vi "LDA_IP_An_mx.vi"(0 "Board type":T1=enum."NI-DAQmx", 1 "interval scanning":bool, 7 "Trigger mode":T2, 9 "output polarity":u16(ring)=1 items=["do not change", "positive", "negative"], 13 "Local Client?":bool=TRUE) -> (3 "LDA Binary output":u16[][](array[numeric]), 6 "I16 TOF block (mu.s)":i16[](array[numeric])=[-338, -324, -346, -351, -326, -357, -344, -311, -375, -296], 15 "error out":errorcluster)   [LabVIEW 2011]
uses:
  Controls/Trigger_Mode.ctl
  Controls/Board_Types.ctl
  Controls/Block_start_and_end.ctl
  <vilib>/DAQmx/read.llb/DAQmx Read (Analog 2D DBL NChan NSamp).vi
  Globals/Meas_global.vi
  Globals/LDA_meas_global_1.vi
  PWA/PWAtasksGLOBAL.vi
  <vilib>/DAQmx/configure/timing.llb/DAQmx Timing (Sample Clock).vi
  <vilib>/DAQmx/create/channels.llb/DAQmx Create Channel (AI-Voltage-Basic).vi
  Globals/LDA_meas_global_2.vi
  <vilib>/DAQmx/miscellaneous.llb/DAQmx Fill In Error Info.vi
  Program Files/National Instruments/LabVIEW 2011/resource/objmgr/daqmx.rc
panel:
  out "AI.Voltage.Rngs":dbl[](array[numeric])=[-10.0, 10.0]
  out "TotalSampPerChanAcquired":dbl=1024.0
  out "AvailSampPerChan":u32
  out "CurrReadPos":dbl=1024.0
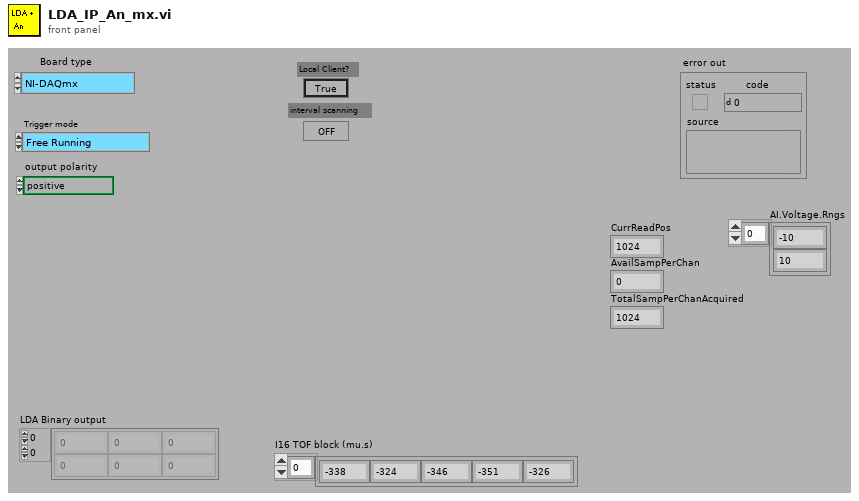
[diagram p1: front panel]
types:
  T1 = typedef "Board_Types.ctl" = enum16{"Simulate", "Local ADAM", "Server ADAM", "NI-DAQmx", "NI-DAQmxBase", "ADC488", "DT LV-link"}
  T2 = typedef "Trigger_Mode.ctl" = enum16{"Free Running", "Start on Trigger", "Trigger Every Block", "Trigger Every Sample"}
  T3 = typedef "Ch_and_Spans.ctl" = cluster{"high limit (10V)":sgl, "low limit (-10V)":sgl, "Ch No":i16, "Var name":string, "Use Latest Calib":bool}
  T4 = typedef "Block_start_and_end.ctl" = cluster{"Started":dbl, "Ended":dbl, "Analogue Frequency Hz":dbl}
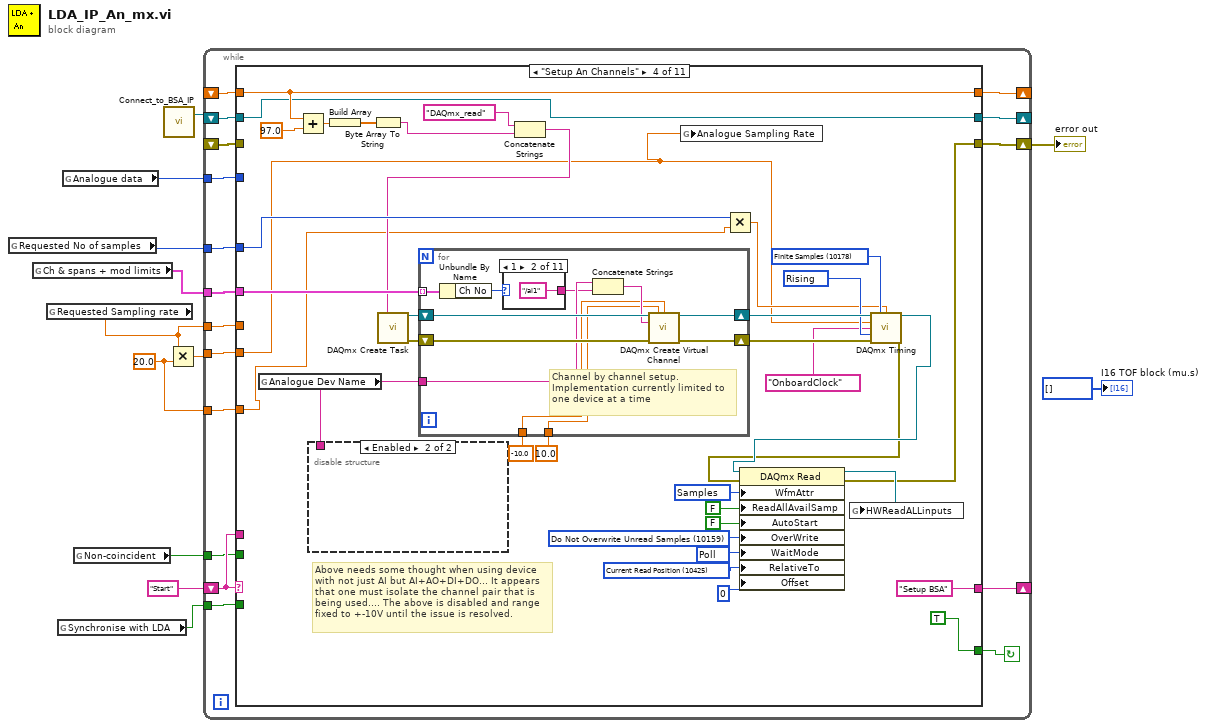
[diagram p0: block diagram]
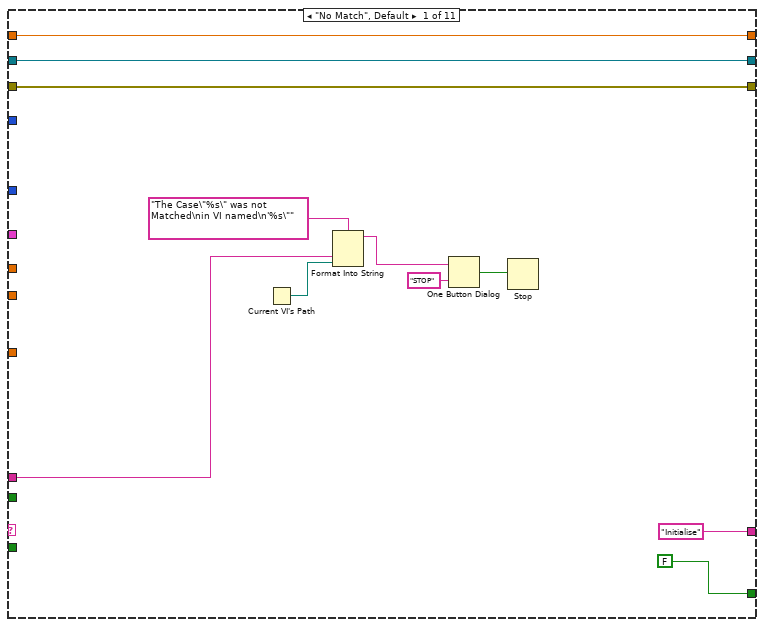
[diagram p2: hidden frame]
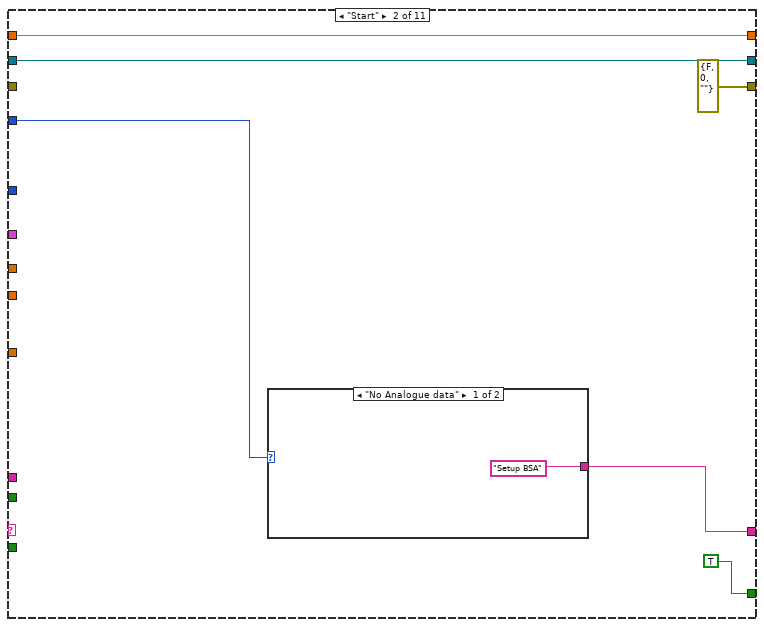
[diagram p3: hidden frame]
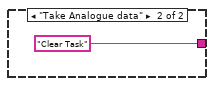
[diagram p4: hidden frame]
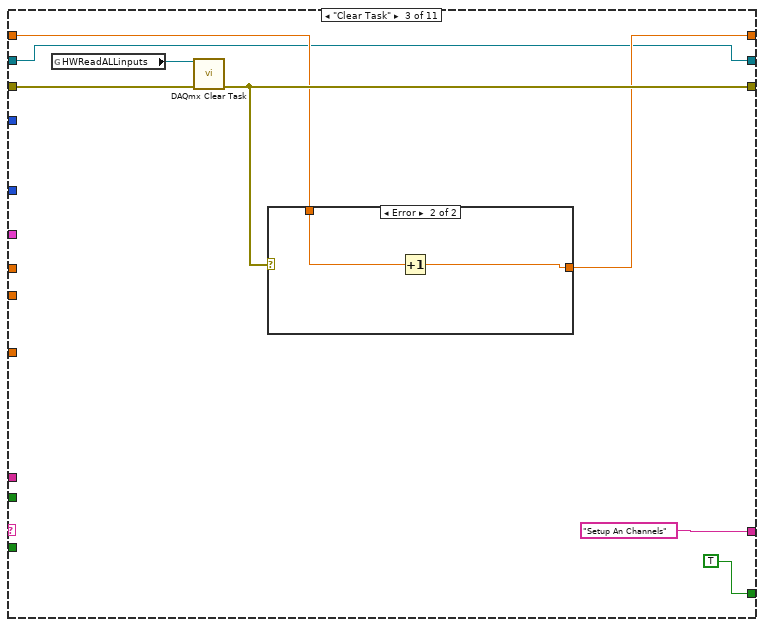
[diagram p5: hidden frame]
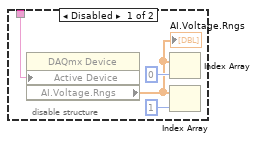
[diagram p7: hidden frame]
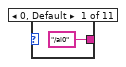
[diagram p8: hidden frame]
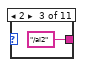
[diagram p9: hidden frame]
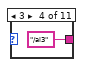
[diagram p10: hidden frame]
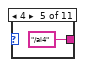
[diagram p11: hidden frame]
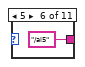
[diagram p12: hidden frame]
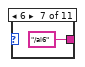
[diagram p13: hidden frame]
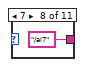
[diagram p14: hidden frame]
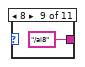
[diagram p15: hidden frame]
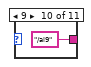
[diagram p16: hidden frame]
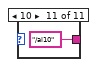
[diagram p17: hidden frame]
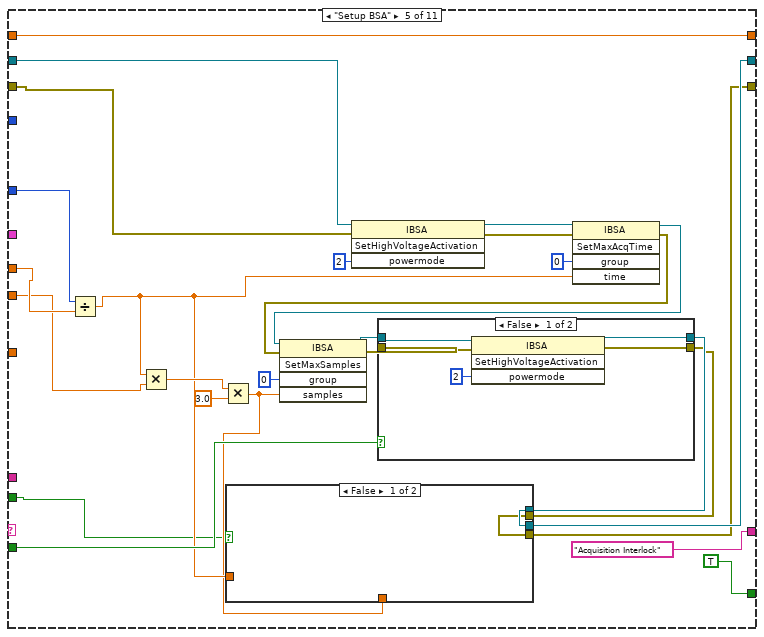
[diagram p18: hidden frame]
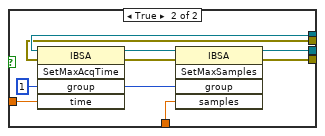
[diagram p19: hidden frame]
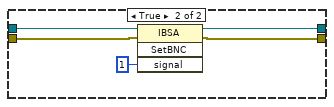
[diagram p20: hidden frame]
diagram:
  w8 = 20.0 ("y")
  n1 = global read "Meas_global.vi" "Requested No of samples"() -> (w1:i32)
  n2 = global read "Meas_global.vi" "Ch & spans + mod limits"() -> (w3:T3[])
  n3 = global read "Meas_global.vi" "Requested Sampling rate"() -> (w2:dbl)
  n4 = global read "Meas_global.vi" "Synchronise with LDA"() -> (w5:bool)
  n5 = global read "Meas_global.vi" "Analogue data"() -> (w6:enum16{"No Analogue data", "Take Analogue data"})
  n6 = global read "LDA_meas_global_1.vi" "Non-coincident"() -> (w4:bool)
  n7 = call "Connect_to_BSA_IP.vi"() -> ("BSA"=w7:refnum<k7>)  [unwired: 3 out]
  n8 = Multiply(x=w2, y=w8) -> (x*y=w9:dbl)
  n9 = while {
    shift-left: "Start" -> [w27]
    shift-right: [w28] -> _
    shift-right: [w22] -> w11
    shift-left: _ -> [w26]
    tunnel: w9 -> [w25]
    tunnel: w1 -> [w24]
    tunnel: w3 -> [w23]
    shift-right: [w21] -> _
    shift-left: _ -> [w20]
    tunnel: w2 -> [w19]
    tunnel: w8 -> [w18]
    shift-right: [w16] -> _
    shift-left: w7 -> [w17]
    tunnel: w6 -> [w15]
    tunnel: w5 -> [w14]
    tunnel: w4 -> [w13]
    stop <- w29 continue-if-true
    n10 = case shown="\"Setup An Channels\"" w27 {
      tunnel: [FALSE TRUE TRUE TRUE TRUE TRUE TRUE w220 w297 FALSE FALSE] -> w29
      tunnel: ["Initialise" w44 "Setup An Channels" "Setup BSA" "Acquisition Interlock" "Start Task" w177 w241 w300 "End" "End" ("f")] -> w28
      tunnel: w27 -> [w35 _ _ _ _ _ _ _ _ _ _]
      tunnel: [w32 errorcluster {"status"=FALSE, "code"=0, "source"=""} ("error out") w52 w61 w125 w173 w191 w218 w266 w316 w325] -> w22
      tunnel: w26 -> [w32 _ w53 _ w135 w173 w179 w219 w264 w322 w325]
      tunnel: w25 -> [_ _ _ w60 w136 _ w187 _ _ _ _]
      tunnel: w24 -> [_ _ _ w87 w138 _ w189 _ _ w307 _]
      tunnel: w23 -> [_ _ _ w90 _ _ _ _ _ _ _]
      tunnel: [w31 w42 w51 w75 w134 w171 w192 w240 w299 w311 w324] -> w21
      tunnel: w20 -> [w31 w42 w50 w75 w134 w171 w192 w240 w299 w311 w324]
      tunnel: w19 -> [_ _ _ _ w137 _ w188 _ _ _ _]
      tunnel: w18 -> [_ _ _ w74 _ _ _ _ _ w310 _]
      tunnel: w17 -> [w30 w46 w49 w73 w139 w170 w185 w226 w265 w308 w323]
      tunnel: [w30 w46 w49 w73 w127 w170 w184 w214 w263 w308 w323] -> w16
      tunnel: w15 -> [_ w45 _ _ _ _ w178 w221 w298 _ _]
      tunnel: w14 -> [_ _ _ _ w129 _ _ _ _ _ _]
      tunnel: w13 -> [_ _ _ _ w122 _ w176 _ _ _ _]
      frame "No Match", Default {
        n11 = Current VI's Path() -> (path=w34:path)
        n12 = Format Into String(format string="The Case\"%s\" was not Matched\nin VI named\n'%s\"" ("Format String"), w35, w34) -> (resulting string=w38:string)  [unwired: 2 in, 1 out]
        n13 = One Button Dialog(message=w38, button name ("OK")="STOP") -> (true=w36:bool)
        n14 = Stop(stop? (T)=w36) -> ()
      }
      frame "Start" {
        n15 = case shown="\"No Analogue data\"" w45 {
          tunnel: ["Setup BSA" "Clear Task"] -> w44
          frame "No Analogue data" {
          }
          frame "Take Analogue data" {
          }
        }
      }
      frame "Clear Task" {
        n16 = global read "PWAtasksGLOBAL.vi" "HWReadALLinputs"() -> (w54:refnum<k21>)
        n17 = call <vilib>:"DAQmx Clear Task.vi"("task in"=w54, "error in"=w53) -> ("error out"=w52:errorcluster)  [unwired: 13 out]
        n18 = case shown="Error" w52 {
          tunnel: [w57 w58] -> w51
          tunnel: w50 -> [w57 w59]
          frame No Error {
          }
          frame Error {
            n19 = Increment(x=w59) -> (x+1=w58:dbl)
          }
        }
      }
      frame "Setup An Channels" {
        w66 = 10425 items=["First Sample"=10424, "Current Read Position"=10425, "Reference Trigger"=10426, "First Pretrigger Sample"=10427, "Most Recent Sample"=10428] ("RelativeTo")
        w67 = 12524 items=["Wait For Interrupt"=12523, "Poll"=12524, "Yield"=12525, "Sleep"=12547] ("WaitMode")
        w68 = 10159 items=["Overwrite Unread Samples"=10252, "Do Not Overwrite Unread Samples"=10159] ("OverWrite")
        w70 = 10287 items=["Samples"=10287, "Samples and Timing"=10140, "Samples, Timing, and Attributes"=10141] ("WfmAttr")
        w89 = 10280 items=["Rising"=10280, "Falling"=10171] ("active edge")
        w93 = 10178 items=["Finite Samples"=10178, "Continuous Samples"=10123, "Hardware Timed Single Point"=12522] ("sample mode")
        # "Above needs some thought when using device with not just AI but AI+AO+DI+DO... It appears that one must isolate the channel pair that is being used.... The above is disabled and range fixed to +-10V until the issue is resolved."
        n20 = global read "PWAtasksGLOBAL.vi" "Analogue Dev Name"() -> (w82:string)
        n21 = Add(x=w75, y=97.0) -> (x+y=w80:dbl)
        n22 = disable-structure shown="Enabled" {
          disable-tunnel: w82 -> [w96 _]
          frame Disabled {
            n23 = property class="DAQmx Device"("Active Device"=w96) -> ("AI.Voltage.Rngs"=w97:dbl[])  [unwired: 2 in, 2 out]
            "AI.Voltage.Rngs" <- w97
            n24 = Index Array(array=w97, index=0) -> ()  [unwired: 1 out]
            n25 = Index Array(array=w97, index=1) -> ()  [unwired: 1 out]
          }
          frame Enabled {
          }
        }
        n26 = Build Array(w80) -> (w79:dbl[])
        n27 = Byte Array To String(unsigned byte array=w79) -> (string=w77:string)
        n28 = Concatenate Strings("DAQmx_read" ("new task name"), w77) -> (w76:string)
        n29 = call <vilib>:"DAQmx Create Task.vi"("new task name"=w76) -> ("task out"=w91:refnum<k21>, "error out"=w94:errorcluster)  [unwired: 4 in, 9 out]
        n30 = for {
          tunnel: w90 -> [w110] mode=indexing
          shift-right: [w108] -> w92
          shift-left: w91 -> [w109]
          shift-right: [w106] -> w95
          shift-left: w94 -> [w107]
          tunnel: w82 -> [w104]
          tunnel: -10.0 -> [w101]
          tunnel: 10.0 -> [w100]
          # "Channel by channel setup. Implementation currently limited to one device at a time"
          n31 = Unbundle By Name(w110) -> ("Ch No"=w105:i16)
          n32 = case shown="1" w105 {
            tunnel: ["/ai0" ("string") "/ai1" ("string") "/ai2" ("string") "/ai3" ("string") "/ai4" ("string") "/ai5" ("string") "/ai6" ("string") "/ai7" ("string") "/ai8" ("string") "/ai9" ("string") "/ai10" ("string")] -> w103
            frame 0, Default {
            }
            frame 1 {
            }
            frame 2 {
            }
            frame 3 {
            }
            frame 4 {
            }
            frame 5 {
            }
            frame 6 {
            }
            frame 7 {
            }
            frame 8 {
            }
            frame 9 {
            }
            frame 10 {
            }
          }
          n33 = Concatenate Strings(w104, w103) -> (w102:string)
          n34 = call-poly <vilib>:"DAQmx Create Virtual Channel.vi"("task in"=w109, "maximum value"=w100, "minimum value"=w101, "physical channels"=w102, "error in"=w107) -> ("task out"=w108:refnum<k21>, "error out"=w106:errorcluster)  [unwired: 4 in, 5 out]
        }
        n35 = global write "Meas_global.vi" "Analogue Sampling Rate"(w60) -> ()
        n36 = Multiply(x=w87, y=w74) -> (x*y=w86:dbl)
        n37 = call-poly <vilib>:"DAQmx Timing.vi"("task/channels in"=w92, "sample mode"=w93, "samples per channel"=w86, "rate"=w60, "source"=tag "OnboardClock", "active edge"=w89, "error in"=w95) -> ("task out"=w64:refnum<k21>, "error out"=w62:errorcluster)  [unwired: 7 out]
        n38 = property class="DAQmx Read"(reference=w64, error in=w62, "WfmAttr"=w70, "ReadAllAvailSamp"=FALSE, "AutoStart"=FALSE, "OverWrite"=w68, "WaitMode"=w67, "RelativeTo"=w66, "Offset"=0) -> (reference out=w63:refnum<k21>, error out=w61:errorcluster)
        n39 = global write "PWAtasksGLOBAL.vi" "HWReadALLinputs"(w63) -> ()
      }
      frame "Setup BSA" {
        n40 = Divide(x=w138, y=w137) -> (x/y=w124:dbl)
        n41 = Multiply(x=w124, y=w136) -> (x*y=w140:dbl)
        n42 = Multiply(x=w140, y=3.0) -> (x*y=w123:dbl)
        n43 = invoke class="IBSA" method="SetHighVoltageActivation"(reference=w139, error in=w135, "powermode"=2) -> (reference out=w146:refnum<k7>, error out=w148:errorcluster)  [unwired: 1 in, 2 out]
        n44 = invoke class="IBSA" method="SetMaxAcqTime"(reference=w146, error in=w148, "group"=0, "time"=w124) -> (reference out=w147:refnum<k7>, error out=w145:errorcluster)  [unwired: 1 in, 3 out]
        n45 = invoke class="IBSA" method="SetMaxSamples"(reference=w147, error in=w145, "group"=0, "samples"=w123) -> (reference out=w131:refnum<k7>, error out=w130:errorcluster)  [unwired: 1 in, 3 out]
        n46 = case shown="False" w129 {
          tunnel: w131 -> [w163 w168]
          tunnel: w130 -> [w162 w167]
          tunnel: [w161 w166] -> w128
          tunnel: [w160 w165] -> w126
          frame False {
            n47 = invoke class="IBSA" method="SetHighVoltageActivation"(reference=w163, error in=w162, "powermode"=2) -> (reference out=w161:refnum<k7>, error out=w160:errorcluster)  [unwired: 1 in, 2 out]
          }
          frame True {
            n48 = invoke class="IBSA" method="SetBNC"(reference=w168, error in=w167, "signal"=1) -> (reference out=w166:refnum<k7>, error out=w165:errorcluster)  [unwired: 1 in, 2 out]
          }
        }
        n49 = case shown="False" w122 {
          tunnel: w128 -> [w150 w157]
          tunnel: [w150 w155] -> w127
          tunnel: w126 -> [w149 w154]
          tunnel: [w149 w153] -> w125
          tunnel: w124 -> [_ w152]
          tunnel: w123 -> [_ w151]
          frame False {
          }
          frame True {
            w158 = 1 ("group")
            n50 = invoke class="IBSA" method="SetMaxAcqTime"(reference=w157, error in=w154, "group"=w158, "time"=w152) -> (reference out=w156:refnum<k7>, error out=w159:errorcluster)  [unwired: 1 in, 3 out]
            n51 = invoke class="IBSA" method="SetMaxSamples"(reference=w156, error in=w159, "group"=w158, "samples"=w151) -> (reference out=w155:refnum<k7>, error out=w153:errorcluster)  [unwired: 1 in, 3 out]
          }
        }
      }
      frame "Acquisition Interlock" {
        n52 = call "Acquisition_Interlock.vi"("Local Control"="Local Client?") -> ()
      }
      frame "Start Task" {
        n53 = Divide(x=w189, y=w188) -> (x/y=w186:dbl)
        n54 = global read "PWAtasksGLOBAL.vi" "HWReadALLinputs"() -> (w180:refnum<k21>)
        n55 = Multiply(x=w186, y=w187) -> (x*y=w183:dbl)
        n56 = Multiply(x=w183, y=3.0) -> (x*y=w182:dbl)
        n57 = case shown="\"Take Analogue data\"" w178 {
          tunnel: w179 -> [w199 w206]
          tunnel: [w198 w204] -> w191
          tunnel: w180 -> [w200 w208]
          tunnel: [w200 w207] -> w190
          tunnel: w186 -> [_ _]
          tunnel: w182 -> [_ _]
          tunnel: w185 -> [w196 w205]
          tunnel: [w197 w203] -> w184
          frame "No Analogue data" {
            n58 = invoke class="IBSA" method="StartAcq"(reference=w196, error in=w199, "waitAcqDone"=1) -> (reference out=w197:refnum<k7>, error out=w198:errorcluster)  [unwired: 1 in, 2 out]
          }
          frame "Take Analogue data" {
            n59 = stacked-sequence {
              tunnel: w208 -> [_ w211]
              tunnel: [_ w210] -> w207
              frame #0 {
                n60 = Wait (ms)(milliseconds to wait=u32 600) -> ()  [unwired: 1 out]
              }
              frame #1 {
                n61 = call <vilib>:"DAQmx Start Task.vi"("task/channels in"=w211) -> ("task out"=w210:refnum<k21>)  [unwired: 1 in, 13 out]
              }
            }
            n62 = invoke class="IBSA" method="StartAcq"(reference=w205, error in=w206, "waitAcqDone"=1) -> (reference out=w203:refnum<k7>, error out=w204:errorcluster)  [unwired: 1 in, 2 out]
          }
        }
        n63 = case shown="True" w176 {
          tunnel: ["Get LDA Data" "Get LDA data Non-coincident"] -> w177
          frame False {
          }
          frame True {
          }
        }
        n64 = global write "PWAtasksGLOBAL.vi" "HWReadALLinputs"(w190) -> ()
      }
      frame "Get LDA Data" {
        w234 = dbl[] []  # Array Constant
        w222 = 0 ("group")
        n65 = invoke class="IBSA" method="ReadArrivalTimeData"(reference=w226, error in=w219, "group"=w222) -> (reference out=w239:refnum<k7>, error out=w238:errorcluster, "ReadArrivalTimeData"=w233:variant)  [unwired: 1 in, 1 out]
        n66 = global read "Meas_global.vi" "dimensions"() -> (w223:enum16{"1D", "2D"})
        n67 = invoke class="IBSA" method="ReadTransitTimeData"(reference=w239, error in=w238, "group"=w222) -> (reference out=w237:refnum<k7>, error out=w236:errorcluster, "ReadTransitTimeData"=w232:variant)  [unwired: 1 in, 1 out]
        n68 = invoke class="IBSA" method="ReadVelocityData"(reference=w237, error in=w236, "group"=w222, "channel"=0) -> (reference out=w225:refnum<k7>, error out=w224:errorcluster, "ReadVelocityData"=w231:variant)  [unwired: 1 in, 2 out]
        n69 = case shown="\"2D\"" w223 {
          tunnel: w234 -> [w248 w257]
          tunnel: [w248 w255] -> w227
          tunnel: [w249 w254] -> w214
          tunnel: w225 -> [w249 w253]
          tunnel: w224 -> [w247 w252]
          tunnel: w222 -> [_ w251]
          tunnel: [w247 w250] -> w218
          frame "1D" {
          }
          frame "2D" {
            n70 = invoke class="IBSA" method="ReadVelocityData"(reference=w253, error in=w252, "group"=w251, "channel"=1) -> (reference out=w254:refnum<k7>, error out=w250:errorcluster, "ReadVelocityData"=w256:variant)  [unwired: 1 in, 2 out]
            n71 = Variant To Data(type=w257, Variant=w256) -> (data=w255:dbl[])  [unwired: 1 in, 1 out]
          }
        }
        n72 = case shown="\"No Analogue data\"" w221 {
          tunnel: ["End" "Read An data"] -> w241
          tunnel: [FALSE TRUE] -> w220
          frame "No Analogue data" {
          }
          frame "Take Analogue data" {
          }
        }
        n73 = Variant To Data(type=w234, Variant=w233) -> (data=w230:dbl[])  [unwired: 1 in, 1 out]
        n74 = Variant To Data(type=w234, Variant=w232) -> (data=w229:dbl[])  [unwired: 1 in, 1 out]
        n75 = Variant To Data(type=w234, Variant=w231) -> (data=w228:dbl[])  [unwired: 1 in, 1 out]
        n76 = Build Array(w230, w229, w228, w227) -> (w212:dbl[][])
        n77 = global write "LDA_meas_global_2.vi" "LDA 1st Group"(w212) -> ()
        n78 = Array Size(array=w212) -> (size(s)=w217:i32[])
        n79 = Index Array(array=w217, index=0) -> (element=w215:i32)
        n80 = Equal To 0?(x=w215) -> (x = 0?=w213:bool)
        n81 = case shown="True" w213 {
          tunnel: w214 -> [_ w242]
          frame False {
          }
          frame True {
            n82 = invoke class="IBSA" method="Disconnect"(reference=w242) -> ()  [unwired: 2 in, 3 out]
          }
        }
      }
      frame "Get LDA data Non-coincident" {
        w273 = dbl[] []  # Array Constant
        w280 = 1 ("group")
        w287 = dbl[] []  # Array Constant
        w281 = 0 ("group")
        n83 = invoke class="IBSA" method="ReadArrivalTimeData"(reference=w265, error in=w264, "group"=w281) -> (reference out=w292:refnum<k7>, error out=w291:errorcluster, "ReadArrivalTimeData"=w286:variant)  [unwired: 1 in, 1 out]
        n84 = invoke class="IBSA" method="ReadTransitTimeData"(reference=w292, error in=w291, "group"=w281) -> (reference out=w290:refnum<k7>, error out=w289:errorcluster, "ReadTransitTimeData"=w285:variant)  [unwired: 1 in, 1 out]
        n85 = invoke class="IBSA" method="ReadVelocityData"(reference=w290, error in=w289, "group"=w281, "channel"=0) -> (reference out=w267:refnum<k7>, error out=w268:errorcluster, "ReadVelocityData"=w284:variant)  [unwired: 1 in, 2 out]
        n86 = invoke class="IBSA" method="ReadArrivalTimeData"(reference=w267, error in=w268, "group"=w280) -> (reference out=w275:refnum<k7>, error out=w276:errorcluster, "ReadArrivalTimeData"=w269:variant)  [unwired: 1 in, 1 out]
        n87 = invoke class="IBSA" method="ReadTransitTimeData"(reference=w275, error in=w276, "group"=w280) -> (reference out=w277:refnum<k7>, error out=w278:errorcluster, "ReadTransitTimeData"=w270:variant)  [unwired: 1 in, 1 out]
        n88 = invoke class="IBSA" method="ReadVelocityData"(reference=w277, error in=w278, "group"=w280, "channel"=1) -> (reference out=w263:refnum<k7>, error out=w266:errorcluster, "ReadVelocityData"=w271:variant)  [unwired: 1 in, 2 out]
        n89 = case shown="\"No Analogue data\"" w298 {
          tunnel: ["End" "Read An data"] -> w300
          tunnel: [FALSE TRUE] -> w297
          frame "No Analogue data" {
          }
          frame "Take Analogue data" {
          }
        }
        n90 = Variant To Data(type=w273, Variant=w269) -> (data=w274:dbl[])  [unwired: 1 in, 1 out]
        n91 = Variant To Data(type=w273, Variant=w270) -> (data=w272:dbl[])  [unwired: 1 in, 1 out]
        n92 = Variant To Data(type=w273, Variant=w271) -> (data=w260:dbl[])  [unwired: 1 in, 1 out]
        n93 = Variant To Data(type=w287, Variant=w286) -> (data=w283:dbl[])  [unwired: 1 in, 1 out]
        n94 = Variant To Data(type=w287, Variant=w285) -> (data=w282:dbl[])  [unwired: 1 in, 1 out]
        n95 = Variant To Data(type=w287, Variant=w284) -> (data=w261:dbl[])  [unwired: 1 in, 1 out]
        n96 = Build Array(w274, w272, w260) -> (w262:dbl[][])
        n97 = global write "LDA_meas_global_2.vi" "LDA 2nd Group"(w262) -> ()
        n98 = Build Array(w283, w282, w261) -> (w259:dbl[][])
        n99 = Array Size(array=w259) -> (size(s)=w296:i32[])
        n100 = global write "LDA_meas_global_2.vi" "LDA 1st Group"(w259) -> ()
        n101 = Index Array(array=w296, index=0) -> (element=w294:i32)
        n102 = Equal To 0?(x=w294) -> (x = 0?=w293:bool)
        n103 = case shown="True" w293 {
          tunnel: w263 -> [_ w301]
          frame False {
          }
          frame True {
            n104 = invoke class="IBSA" method="Disconnect"(reference=w301) -> ()  [unwired: 2 in, 3 out]
          }
        }
      }
      frame "Read An data" {
        n105 = global read "PWAtasksGLOBAL.vi" "HWReadALLinputs"() -> (w314:refnum<k21>)
        n106 = Multiply(x=w307, y=w310) -> (x*y=w309:dbl)
        n107 = call-poly <vilib>:"DAQmx Read.vi"("task/channels in"=w314, "number of samples per channel"=w309, "error in"=w322) -> ("task out"=w319:refnum<k21>, "data"=w306:dbl[][], "error out"=w313:errorcluster)  [unwired: 10 out]
        n108 = property class="DAQmx Read"(reference=w319, error in=w313) -> (reference out=w318:refnum<k21>, error out=w316:errorcluster, "CurrReadPos"=→"CurrReadPos":dbl, "AvailSampPerChan"=→"AvailSampPerChan":u32, "TotalSampPerChanAcquired"=→"TotalSampPerChanAcquired":dbl)
        n109 = global write "PWAtasksGLOBAL.vi" "HWReadALLinputs"(w318) -> ()
        n110 = global write "Meas_global.vi" "Analogue volts"(w306) -> ()
      }
      frame "Extra case" {
        (unwired) T4 {"Started"=0.0, "Ended"=0.0, "Analogue Frequency Hz"=1000.0} ("Block Timings")
      }
    }
  }
  "error out" <- w11
  "I16 TOF block (mu.s)" <- i16[] [] ("I16 TOF block (mu.s)")
